vi "RegisterWithNode.vi"(0 "ROS":T3={"topic port"=0, "Node"="", "topic"="", "type"="", "node port"=0, "error "={"status"=FALSE, "code"=0, "source"=""}, "Direction"=enum."Node", "APIs"=[], "Update (ms)"=1, "write queue"=1}) -> (1 "MyState":T2, 2 "Log":T1)   [LabVIEW 2012]
uses:
  <userlib>/ROSforLV/ROS/Code/SubVIs/_ROSControl.ctl
  <userlib>/ROSforLV/ROS/Code/SubVIs/_ROSDirection.ctl
  <userlib>/ROSforLV/ROS/Code/Console/Servers/ServerSubs/MyState.ctl
  <userlib>/ROSforLV/ROS/Code/Console/Servers/ServerSubs/ROSLog.ctl
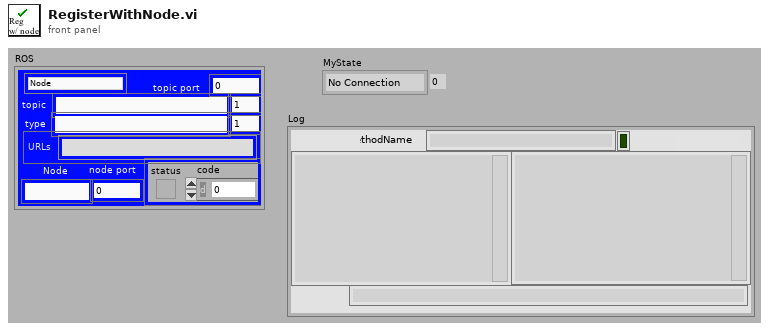
[diagram p1: front panel]
types:
  T1 = typedef "ROSLog.ctl" = cluster{"Sent":string, "Reply":string, "MethodName":string, "success":bool, "Dir1":string, "Dir2":string, "Time Stamp":string, "error":errorcluster, "Preamble":string, "Midamble":string, "Postamble":string}
  T2 = typedef "MyState.ctl" = enum16{"No Connection", "Registered", "Connected", "Close"}
  T3 = typedef "_ROSControl.ctl" = cluster{"topic port":u16, "Node":string, "topic":string, "type":string, "node port":u16, "error ":errorcluster, "Direction":T4, "APIs":string[], "Update (ms)":u16, "write queue":u16}
  T4 = typedef "_ROSDirection.ctl" = enum16{"Node", "Publisher", "Subscriber", "Service Client"}
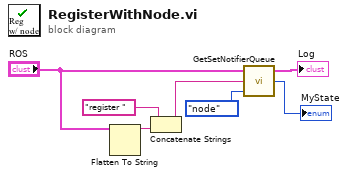
[diagram p0: block diagram]
diagram:
  n1 = Flatten To String(anything="ROS") -> (data string=w5:string)  [unwired: 3 in, 2 out]
  n2 = Concatenate Strings("register " ("Command"), w5) -> (w3:string)
  n3 = call <userlib>:"GetSetNotifierQueue.vi"("Name"=enum16{"topic", "node"}."node", "Command"=w3, "ROS"="ROS") -> ("MyState"=→"MyState":T2, "Log"=→"Log":T1)  [unwired: 1 in]
